vi "GeoData.vi"() -> ()   [LabVIEW 2017] (continued)
davenport\tNY\tDelaware County\tH1\n12468\t36025\tPrattsville\tNY\tDelaware County\tH1\n12760\t36025\tLong eddy\tNY\tDelaware County\tH1\n13820\t36025\tOneonta\tNY\tDelaware County\tH1\n13775\t36025\tFranklin\tNY\tDelaware County\tH1\n12430\t36025\tFleischmanns\tNY\tDelaware County\tH1\n12533\t36027\tHopewell junction\tNY\tDutchess County\tH1\n12545\t36027\tMillbrook\tNY\tDutchess County\tH1\n12583\t36027\tTivoli\tNY\tDutchess County\tH1\n12527\t36027\tGlenham\tNY\tDutchess County\tH1\n10512\t36027\tCarmel\tNY\tDutchess County\tH1\n12569\t36027\tPleasant valley\tNY\tDutchess County\tH1\n12601\t36027\tPoughkeepsie\tNY\tDutchess County\tH1\n12603\t36027\tPoughkeepsie\tNY\tDutchess County\tH1\n12511\t36027\tCastle point\tNY\tDutchess County\tH1\n12507\t36027\tBarrytown\tNY\tDutchess County\tH1\n12564\t36027\tPawling\tNY\tDutchess County\tH1\n12602\t36027\tPoughkeepsie\tNY\tDutchess County\tH1\n12531\t36027\tHolmes\tNY\tDutchess County\tH1\n12572\t36027\tRhinebeck\tNY\tDutchess County\tH1\n12538\t36027\tHyde park\tNY\tDutchess County\tH1\n12571\t36027\tRed hook\tNY\tDutchess County\tH1\n12594\t36027\tWingdale\tNY\tDutchess County\tH1\n12501\t36027\tAmenia\tNY\tDutchess County\tH1\n12570\t36027\tPoughquag\tNY\tDutchess County\tH1\n12581\t36027\tStanfordville\tNY\tDutchess County\tH1\n12582\t36027\tStormville\tNY\tDutchess County\tH1\n12590\t36027\tWappingers falls\tNY\tDutchess County\tH1\n12580\t36027\tStaatsburg\tNY\tDutchess County\tH1\n12546\t36027\tMillerton\tNY\tDutchess County\tH1\n12508\t36027\tBeacon\tNY\tDutchess County\tH1\n12540\t36027\tLagrangeville\tNY\tDutchess County\tH1\n12522\t36027\tDover plains\tNY\tDutchess County\tH1\n12504\t36027\tAnnandale on hudson\tNY\tDutchess County\tH1\n12537\t36027\tHughsonville\tNY\tDutchess County\tH1\n12574\t36027\tRhinecliff\tNY\tDutchess County\tH1\n12524\t36027\tFishkill\tNY\tDutchess County\tH1\n12585\t36027\tVerbank\tNY\tDutchess County\tH1\n12578\t36027\tSalt point\tNY\tDutchess County\tH1\n12567\t36027\tPine plains\tNY\tDutchess County\tH1\n12592\t36027\tWassaic\tNY\tDutchess County\tH1\n12514\t36027\tClinton corners\tNY\tDutchess County\tH1\n12506\t36027\tBangall\tNY\tDutchess County\tH1\n12512\t36027\tChelsea\tNY\tDutchess County\tH1\n12510\t36027\tBillings\tNY\tDutchess County\tH1\n12604\t36027\tPoughkeepsie\tNY\tDutchess County\tH1\n14052\t36029\tEast aurora\tNY\tErie County\tH1\n14036\t36029\tCorfu\tNY\tErie County\tH1\n14210\t36029\tBuffalo\tNY\tErie County\tH1\n14202\t36029\tBuffalo\tNY\tErie County\tH1\n14151\t36029\tTonawanda\tNY\tErie County\tH1\n14213\t36029\tBuffalo\tNY\tErie County\tH1\n14170\t36029\tWest falls\tNY\tErie County\tH1\n14219\t36029\tBuffalo\tNY\tErie County\tH1\n14223\t36029\tBuffalo\tNY\tErie County\tH1\n14085\t36029\tLake view\tNY\tErie County\tH1\n14080\t36029\tHolland\tNY\tErie County\tH1\n14134\t36029\tSardinia\tNY\tErie County\tH1\n14037\t36029\tCowlesville\tNY\tErie County\tH1\n14030\t36029\tChaffee\tNY\tErie County\tH1\n14241\t36029\tBuffalo\tNY\tErie County\tH1\n14059\t36029\tElma\tNY\tErie County\tH1\n14221\t36029\tBuffalo\tNY\tErie County\tH1\n14055\t36029\tEast concord\tNY\tErie County\tH1\n14272\t36029\tBuffalo\tNY\tErie County\tH1\n14140\t36029\tSpring brook\tNY\tErie County\tH1\n14075\t36029\tHamburg\tNY\tErie County\tH1\n14057\t36029\tEden\tNY\tErie County\tH1\n14208\t36029\tBuffalo\tNY\tErie County\tH1\n14214\t36029\tBuffalo\tNY\tErie County\tH1\n14206\t36029\tBuffalo\tNY\tErie County\tH1\n14139\t36029\tSouth wales\tNY\tErie County\tH1\n14209\t36029\tBuffalo\tNY\tErie County\tH1\n14225\t36029\tBuffalo\tNY\tErie County\tH1\n14025\t36029\tBoston\tNY\tErie County\tH1\n14260\t36029\tBuffalo\tNY\tErie County\tH1\n14263\t36029\tBuffalo\tNY\tErie County\tH1\n14027\t36029\tBrant\tNY\tErie County\tH1\n14110\t36029\tNorth boston\tNY\tErie County\tH1\n14032\t36029\tClarence center\tNY\tErie County\tH1\n14102\t36029\tMarilla\tNY\tErie County\tH1\n14091\t36029\tLawtons\tNY\tErie County\tH1\n14205\t36029\tBuffalo\tNY\tErie County\tH1\n14240\t36029\tBuffalo\tNY\tErie County\tH1\n14081\t36029\tIrving\tNY\tErie County\tH1\n14203\t36029\tBuffalo\tNY\tErie County\tH1\n14226\t36029\tBuffalo\tNY\tErie County\tH1\n14231\t36029\tBuffalo\tNY\tErie County\tH1\n14280\t36029\tBuffalo\tNY\tErie County\tH1\n14270\t36029\tBuffalo\tNY\tErie County\tH1\n14004\t36029\tAlden\tNY\tErie County\tH1\n14051\t36029\tEast amherst\tNY\tErie County\tH1\n14006\t36029\tAngola\tNY\tErie County\tH1\n14086\t36029\tLancaster\tNY\tErie County\tH1\n14127\t36029\tOrchard park\tNY\tErie County\tH1\n14150\t36029\tTonawanda\tNY\tErie County\tH1\n14211\t36029\tBuffalo\tNY\tErie County\tH1\n14227\t36029\tBuffalo\tNY\tErie County\tH1\n14228\t36029\tBuffalo\tNY\tErie County\tH1\n14070\t36029\tGowanda\tNY\tErie County\tH1\n14145\t36029\tStrykersville\tNY\tErie County\tH1\n14026\t36029\tBowmansville\tNY\tErie County\tH1\n14265\t36029\tBuffalo\tNY\tErie County\tH1\n14112\t36029\tNorth evans\tNY\tErie County\tH1\n14035\t36029\tCollins center\tNY\tErie County\tH1\n14233\t36029\tBuffalo\tNY\tErie County\tH1\n14043\t36029\tDepew\tNY\tErie County\tH1\n14212\t36029\tBuffalo\tNY\tErie County\tH1\n14169\t36029\tWales center\tNY\tErie County\tH1\n14269\t36029\tBuffalo\tNY\tErie County\tH1\n14072\t36029\tGrand island\tNY\tErie County\tH1\n14009\t36029\tArcade\tNY\tErie County\tH1\n14013\t36029\tBasom\tNY\tErie County\tH1\n14207\t36029\tBuffalo\tNY\tErie County\tH1\n14215\t36029\tBuffalo\tNY\tErie County\tH1\n14201\t36029\tBuffalo\tNY\tErie County\tH1\n14204\t36029\tBuffalo\tNY\tErie County\tH1\n14220\t36029\tBuffalo\tNY\tErie County\tH1\n14222\t36029\tBuffalo\tNY\tErie County\tH1\n14224\t36029\tBuffalo\tNY\tErie County\tH1\n14217\t36029\tBuffalo\tNY\tErie County\tH1\n14034\t36029\tCollins\tNY\tErie County\tH1\n14047\t36029\tDerby\tNY\tErie County\tH1\n14010\t36029\tAthol springs\tNY\tErie County\tH1\n14001\t36029\tAkron\tNY\tErie County\tH1\n14031\t36029\tClarence\tNY\tErie County\tH1\n14068\t36029\tGetzville\tNY\tErie County\tH1\n14111\t36029\tNorth collins\tNY\tErie County\tH1\n14216\t36029\tBuffalo\tNY\tErie County\tH1\n14141\t36029\tSpringville\tNY\tErie County\tH1\n14218\t36029\tBuffalo\tNY\tErie County\tH1\n14033\t36029\tColden\tNY\tErie County\tH1\n14069\t36029\tGlenwood\tNY\tErie County\tH1\n14061\t36029\tFarnham\tNY\tErie County\tH1\n14038\t36029\tCrittenden\tNY\tErie County\tH1\n14276\t36029\tBuffalo\tNY\tErie County\tH1\n14273\t36029\tBuffalo\tNY\tErie County\tH1\n12883\t36031\tTiconderoga\tNY\tEssex County\tH1\n12974\t36031\tPort henry\tNY\tEssex County\tH1\n12936\t36031\tEssex\tNY\tEssex County\tH1\n12996\t36031\tWillsboro\tNY\tEssex County\tH1\n12997\t36031\tWilmington\tNY\tEssex County\tH1\n12942\t36031\tKeene\tNY\tEssex County\tH1\n12998\t36031\tWitherbee\tNY\tEssex County\tH1\n12857\t36031\tOlmstedville\tNY\tEssex County\tH1\n12861\t36031\tPutnam station\tNY\tEssex County\tH1\n12956\t36031\tMineville\tNY\tEssex County\tH1\n12943\t36031\tKeene valley\tNY\tEssex County\tH1\n12983\t36031\tSaranac lake\tNY\tEssex County\tH1\n12993\t36031\tWestport\tNY\tEssex County\tH1\n12941\t36031\tJay\tNY\tEssex County\tH1\n12975\t36031\tPort kent\tNY\tEssex County\tH1\n12855\t36031\tNorth hudson\tNY\tEssex County\tH1\n12836\t36031\tHague\tNY\tEssex County\tH1\n12944\t36031\tKeeseville\tNY\tEssex County\tH1\n12987\t36031\tUpper jay\tNY\tEssex County\tH1\n12961\t36031\tMoriah center\tNY\tEssex County\tH1\n12870\t36031\tSchroon lake\tNY\tEssex County\tH1\n12972\t36031\tPeru\tNY\tEssex County\tH1\n12964\t36031\tNew russia\tNY\tEssex County\tH1\n12911\t36031\tKeeseville\tNY\tEssex County\tH1\n12879\t36031\tNewcomb\tNY\tEssex County\tH1\n12852\t36031\tNewcomb\tNY\tEssex County\tH1\n12946\t36031\tLake placid\tNY\tEssex County\tH1\n12853\t36031\tNorth creek\tNY\tEssex County\tH1\n12928\t36031\tCrown point\tNY\tEssex County\tH1\n12851\t36031\tMinerva\tNY\tEssex County\tH1\n12913\t36031\tBloomingdale\tNY\tEssex County\tH1\n12872\t36031\tSeverance\tNY\tEssex County\tH1\n12977\t36031\tRay brook\tNY\tEssex County\tH1\n12858\t36031\tParadox\tNY\tEssex County\tH1\n12950\t36031\tLewis\tNY\tEssex County\tH1\n12960\t36031\tMoriah\tNY\tEssex County\tH1\n12912\t36031\tAu sable forks\tNY\tEssex County\tH1\n12932\t36031\tElizabethtown\tNY\tEssex County\tH1\n12989\t36031\tVermontville\tNY\tEssex County\tH1\n12916\t36033\tBrushton\tNY\tFranklin County\tH1\n12981\t36033\tSaranac\tNY\tFranklin County\tH1\n12980\t36033\tSaint regis falls\tNY\tFranklin County\tH1\n12955\t36033\tLyon mountain\tNY\tFranklin County\tH1\n12976\t36033\tRainbow lake\tNY\tFranklin County\tH1\n12967\t36033\tNorth lawrence\tNY\tFranklin County\tH1\n12939\t36033\tGabriels\tNY\tFranklin County\tH1\n12926\t36033\tConstable\tNY\tFranklin County\tH1\n12937\t36033\tFort covington\tNY\tFranklin County\tH1\n12914\t36033\tBombay\tNY\tFranklin County\tH1\n12969\t36033\tOwls head\tNY\tFranklin County\tH1\n12953\t36033\tMalone\tNY\tFranklin County\tH1\n12983\t36033\tSaranac lake\tNY\tFranklin County\tH1\n13655\t36033\tHogansburg\tNY\tFranklin County\tH1\n12957\t36033\tMoira\tNY\tFranklin County\tH1\n12966\t36033\tNorth bangor\tNY\tFranklin County\tH1\n13683\t36033\tRooseveltown\tNY\tFranklin County\tH1\n12920\t36033\tChateaugay\tNY\tFranklin County\tH1\n12945\t36033\tLake clear\tNY\tFranklin County\tH1\n12970\t36033\tPaul smiths\tNY\tFranklin County\tH1\n12995\t36033\tWhippleville\tNY\tFranklin County\tH1\n12915\t36033\tBrainardsville\tNY\tFranklin County\tH1\n12930\t36033\tDickinson center\tNY\tFranklin County\tH1\n12913\t36033\tBloomingdale\tNY\tFranklin County\tH1\n12986\t36033\tTupper lake\tNY\tFranklin County\tH1\n12912\t36033\tAu sable forks\tNY\tFranklin County\tH1\n12917\t36033\tBurke\tNY\tFranklin County\tH1\n12989\t36033\tVermontville\tNY\tFranklin County\tH1\n12095\t36035\tJohnstown\tNY\tFulton County\tH1\n13329\t36035\tDolgeville\tNY\tFulton County\tH1\n12086\t36035\tHagaman\tNY\tFulton County\tH1\n12117\t36035\tMayfield\tNY\tFulton County\tH1\n12010\t36035\tAmsterdam\tNY\tFulton County\tH1\n12068\t36035\tFonda\tNY\tFulton County\tH1\n12032\t36035\tCaroga lake\tNY\tFulton County\tH1\n12025\t36035\tBroadalbin\tNY\tFulton County\tH1\n13452\t36035\tSaint johnsville\tNY\tFulton County\tH1\n13470\t36035\tStratford\tNY\tFulton County\tH1\n12070\t36035\tFort johnson\tNY\tFulton County\tH1\n13339\t36035\tFort plain\tNY\tFulton County\tH1\n12078\t36035\tGloversville\tNY\tFulton County\tH1\n12134\t36035\tNorthville\tNY\tFulton County\tH1\n13454\t36035\tSalisbury center\tNY\tFulton County\tH1\n14036\t36037\tCorfu\tNY\tGenesee County\tH1\n14525\t36037\tPavilion\tNY\tGenesee County\tH1\n14005\t36037\tAlexander\tNY\tGenesee County\tH1\n14428\t36037\tChurchville\tNY\tGenesee County\tH1\n14105\t36037\tMiddleport\tNY\tGenesee County\tH1\n14416\t36037\tBergen\tNY\tGenesee County\tH1\n14058\t36037\tElba\tNY\tGenesee County\tH1\n14422\t36037\tByron\tNY\tGenesee County\tH1\n14004\t36037\tAlden\tNY\tGenesee County\tH1\n14020\t36037\tBatavia\tNY\tGenesee County\tH1\n14591\t36037\tWyoming\tNY\tGenesee County\tH1\n14040\t36037\tDarien center\tNY\tGenesee County\tH1\n14557\t36037\tSouth byron\tNY\tGenesee County\tH1\n14103\t36037\tMedina\tNY\tGenesee County\tH1\n14054\t36037\tEast bethany\tNY\tGenesee County\tH1\n14056\t36037\tEast pembroke\tNY\tGenesee County\tH1\n14013\t36037\tBasom\tNY\tGenesee County\tH1\n14125\t36037\tOakfield\tNY\tGenesee County\tH1\n14143\t36037\tStafford\tNY\tGenesee County\tH1\n14482\t36037\tLe roy\tNY\tGenesee County\tH1\n14011\t36037\tAttica\tNY\tGenesee County\tH1\n14021\t36037\tBatavia\tNY\tGenesee County\tH1\n14001\t36037\tAkron\tNY\tGenesee County\tH1\n12413\t36039\tCairo\tNY\tGreene County\tH1\n12485\t36039\tTannersville\tNY\tGreene County\tH1\n12087\t36039\tHannacroix\tNY\tGreene County\tH1\n12450\t36039\tLanesville\tNY\tGreene County\tH1\n12454\t36039\tMaplecrest\tNY\tGreene County\tH1\n12051\t36039\tCoxsackie\tNY\tGreene County\tH1\n12407\t36039\tAshland\tNY\tGreene County\tH1\n12473\t36039\tRound top\tNY\tGreene County\tH1\n12469\t36039\tPreston hollow\tNY\tGreene County\tH1\n12192\t36039\tWest coxsackie\tNY\tGreene County\tH1\n12422\t36039\tDurham\tNY\tGreene County\tH1\n12460\t36039\tOak hill\tNY\tGreene County\tH1\n12015\t36039\tAthens\tNY\tGreene County\tH1\n12427\t36039\tElka park\tNY\tGreene County\tH1\n12176\t36039\tSurprise\tNY\tGreene County\tH1\n12444\t36039\tJewett\tNY\tGreene County\tH1\n12451\t36039\tLeeds\tNY\tGreene County\tH1\n12083\t36039\tGreenville\tNY\tGreene County\tH1\n12058\t36039\tEarlton\tNY\tGreene County\tH1\n12482\t36039\tSouth cairo\tNY\tGreene County\tH1\n12442\t36039\tHunter\tNY\tGreene County\tH1\n12124\t36039\tNew baltimore\tNY\tGreene County\tH1\n12414\t36039\tCatskill\tNY\tGreene County\tH1\n12480\t36039\tShandaken\tNY\tGreene County\tH1\n12042\t36039\tClimax\tNY\tGreene County\tH1\n12418\t36039\tCornwallville\tNY\tGreene County\tH1\n12436\t36039\tHaines falls\tNY\tGreene County\tH1\n12143\t36039\tRavena\tNY\tGreene County\tH1\n12120\t36039\tMedusa\tNY\tGreene County\tH1\n12431\t36039\tFreehold\tNY\tGreene County\tH1\n12492\t36039\tWest kill\tNY\tGreene County\tH1\n12463\t36039\tPalenville\tNY\tGreene County\tH1\n12468\t36039\tPrattsville\tNY\tGreene County\tH1\n12405\t36039\tAcra\tNY\tGreene County\tH1\n12439\t36039\tHensonville\tNY\tGreene County\tH1\n12423\t36039\tEast durham\tNY\tGreene County\tH1\n12430\t36039\tFleischmanns\tNY\tGreene County\tH1\n12470\t36039\tPurling\tNY\tGreene County\tH1\n12046\t36039\tCoeymans hollow\tNY\tGreene County\tH1\n12496\t36039\tWindham\tNY\tGreene County\tH1\n12424\t36039\tEast jewett\tNY\tGreene County\tH1\n12452\t36039\tLexington\tNY\tGreene County\tH1\n13353\t36041\tHoffmeister\tNY\tHamilton County\tH1\n13360\t36041\tInlet\tNY\tHamilton County\tH1\n12864\t36041\tSabael\tNY\tHamilton County\tH1\n12164\t36041\tSpeculator\tNY\tHamilton County\tH1\n12108\t36041\tLake pleasant\tNY\tHamilton County\tH1\n12190\t36041\tWells\tNY\tHamilton County\tH1\n12847\t36041\tLong lake\tNY\tHamilton County\tH1\n12032\t36041\tCaroga lake\tNY\tHamilton County\tH1\n12842\t36041\tIndian lake\tNY\tHamilton County\tH1\n12812\t36041\tBlue mountain lake\tNY\tHamilton County\tH1\n13331\t36041\tEagle bay\tNY\tHamilton County\tH1\n12139\t36041\tPiseco\tNY\tHamilton County\tH1\n12134\t36041\tNorthville\tNY\tHamilton County\tH1\n13436\t36041\tRaquette lake\tNY\tHamilton County\tH1\n13329\t36043\tDolgeville\tNY\tHerkimer County\tH1\n13406\t36043\tMiddleville\tNY\tHerkimer County\tH1\n13360\t36043\tInlet\tNY\tHerkimer County\tH1\n13338\t36043\tForestport\tNY\tHerkimer County\tH1\n13407\t36043\tMohawk\tNY\tHerkimer County\tH1\n13322\t36043\tClayville\tNY\tHerkimer County\tH1\n13420\t36043\tOld forge\tNY\tHerkimer County\tH1\n13413\t36043\tNew hartford\tNY\tHerkimer County\tH1\n13501\t36043\tUtica\tNY\tHerkimer County\tH1\n13361\t36043\tJordanville\tNY\tHerkimer County\tH1\n13340\t36043\tFrankfort\tNY\tHerkimer County\tH1\n13357\t36043\tIlion\tNY\tHerkimer County\tH1\n13456\t36043\tSauquoit\tNY\tHerkimer County\tH1\n13304\t36043\tBarneveld\tNY\tHerkimer County\tH1\n13367\t36043\tLowville\tNY\tHerkimer County\tH1\n13350\t36043\tHerkimer\tNY\tHerkimer County\tH1\n13324\t36043\tCold brook\tNY\tHerkimer County\tH1\n13438\t36043\tRemsen\tNY\tHerkimer County\tH1\n13491\t36043\tWest winfield\tNY\tHerkimer County\tH1\n13431\t36043\tPoland\tNY\tHerkimer County\tH1\n13439\t36043\tRichfield springs\tNY\tHerkimer County\tH1\n13470\t36043\tStratford\tNY\tHerkimer County\tH1\n13502\t36043\tUtica\tNY\tHerkimer County\tH1\n13416\t36043\tNewport\tNY\tHerkimer County\tH1\n13472\t36043\tThendara\tNY\tHerkimer County\tH1\n13339\t36043\tFort plain\tNY\tHerkimer County\tH1\n13365\t36043\tLittle falls\tNY\tHerkimer County\tH1\n13331\t36043\tEagle bay\tNY\tHerkimer County\tH1\n13454\t36043\tSalisbury center\tNY\tHerkimer County\tH1\n13475\t36043\tVan hornesville\tNY\tHerkimer County\tH1\n13145\t36045\tSandy creek\tNY\tJefferson County\tH1\n13601\t36045\tWatertown\tNY\tJefferson County\tH1\n13626\t36045\tCopenhagen\tNY\tJefferson County\tH1\n13619\t36045\tCarthage\tNY\tJefferson County\tH1\n13685\t36045\tSackets harbor\tNY\tJefferson County\tH1\n13636\t36045\tEllisburg\tNY\tJefferson County\tH1\n13671\t36045\tAntwerp\tNY\tJefferson County\tH1\n13693\t36045\tThree mile bay\tNY\tJefferson County\tH1\n13682\t36045\tRodman\tNY\tJefferson County\tH1\n13673\t36045\tPhiladelphia\tNY\tJefferson County\tH1\n13691\t36045\tTheresa\tNY\tJefferson County\tH1\n13606\t36045\tAdams center\tNY\tJefferson County\tH1\n13607\t36045\tAlexandria bay\tNY\tJefferson County\tH1\n13631\t36045\tDenmark\tNY\tJefferson County\tH1\n13622\t36045\tChaumont\tNY\tJefferson County\tH1\n13692\t36045\tThousand island park\tNY\tJefferson County\tH1\n13624\t36045\tClayton\tNY\tJefferson County\tH1\n13616\t36045\tCalcium\tNY\tJefferson County\tH1\n13675\t36045\tPlessis\tNY\tJefferson County\tH1\n13661\t36045\tMannsville\tNY\tJefferson County\tH1\n13602\t36045\tFort drum\tNY\tJefferson County\tH1\n13651\t36045\tHenderson harbor\tNY\tJefferson County\tH1\n13632\t36045\tDepauville\tNY\tJefferson County\tH1\n13615\t36045\tBrownville\tNY\tJefferson County\tH1\n13611\t36045\tBelleville\tNY\tJefferson County\tH1\n13641\t36045\tFishers landing\tNY\tJefferson County\tH1\n13608\t36045\tAntwerp\tNY\tJefferson County\tH1\n13618\t36045\tCape vincent\tNY\tJefferson County\tH1\n13656\t36045\tLa fargeville\tNY\tJefferson County\tH1\n13659\t36045\tLorraine\tNY\tJefferson County\tH1\n13646\t36045\tHammond\tNY\tJefferson County\tH1\n13638\t36045\tFelts mills\tNY\tJefferson County\tH1\n13665\t36045\tNatural bridge\tNY\tJefferson County\tH1\n13634\t36045\tDexter\tNY\tJefferson County\tH1\n13605\t36045\tAdams\tNY\tJefferson County\tH1\n13637\t36045\tEvans mills\tNY\tJefferson County\tH1\n13612\t36045\tBlack river\tNY\tJefferson County\tH1\n13640\t36045\tWellesley island\tNY\tJefferson County\tH1\n13603\t36045\tWatertown\tNY\tJefferson County\tH1\n13642\t36045\tGouverneur\tNY\tJefferson County\tH1\n13650\t36045\tHenderson\tNY\tJefferson County\tH1\n13679\t36045\tRedwood\tNY\tJefferson County\tH1\n13083\t36045\tLacona\tNY\tJefferson County\tH1\n13628\t36045\tDeferiet\tNY\tJefferson County\tH1\n13643\t36045\tGreat bend\tNY\tJefferson County\tH1\n13674\t36045\tPierrepont manor\tNY\tJefferson County\tH1\n11202\t36047\tBrooklyn\tNY\tKings County\tH6\n11204\t36047\tBrooklyn\tNY\tKings County\tH6\n11203\t36047\tBrooklyn\tNY\tKings County\tH6\n11210\t36047\tBrooklyn\tNY\tKings County\tH6\n11213\t36047\tBrooklyn\tNY\tKings County\tH6\n11216\t36047\tBrooklyn\tNY\tKings County\tH6\n11229\t36047\tBrooklyn\tNY\tKings County\tH6\n11225\t36047\tBrooklyn\tNY\tKings County\tH6\n11238\t36047\tBrooklyn\tNY\tKings County\tH6\n11239\t36047\tBrooklyn\tNY\tKings County\tH6\n11211\t36047\tBrooklyn\tNY\tKings County\tH6\n11223\t36047\tBrooklyn\tNY\tKings County\tH6\n11228\t36047\tBrooklyn\tNY\tKings County\tH6\n11417\t36047\tOzone park\tNY\tKings County\tH6\n11242\t36047\tBrooklyn\tNY\tKings County\tH6\n11205\t36047\tBrooklyn\tNY\tKings County\tH6\n11208\t36047\tBrooklyn\tNY\tKings County\tH6\n11212\t36047\tBrooklyn\tNY\tKings County\tH6\n11233\t36047\tBrooklyn\tNY\tKings County\tH6\n11245\t36047\tBrooklyn\tNY\tKings County\tH6\n11206\t36047\tBrooklyn\tNY\tKings County\tH6\n11235\t36047\tBrooklyn\tNY\tKings County\tH6\n11414\t36047\tHoward beach\tNY\tKings County\tH6\n11251\t36047\tBrooklyn\tNY\tKings County\tH6\n11220\t36047\tBrooklyn\tNY\tKings County\tH6\n11247\t36047\tBrooklyn\tNY\tKings County\tH6\n11219\t36047\tBrooklyn\tNY\tKings County\tH6\n11232\t36047\tBrooklyn\tNY\tKings County\tH6\n11236\t36047\tBrooklyn\tNY\tKings County\tH6\n11209\t36047\tBrooklyn\tNY\tKings County\tH6\n11215\t36047\tBrooklyn\tNY\tKings County\tH6\n11214\t36047\tBrooklyn\tNY\tKings County\tH6\n11221\t36047\tBrooklyn\tNY\tKings County\tH6\n11230\t36047\tBrooklyn\tNY\tKings County\tH6\n11234\t36047\tBrooklyn\tNY\tKings County\tH6\n11249\t36047\tBrooklyn\tNY\tKings County\tH6\n11421\t36047\tWoodhaven\tNY\tKings County\tH6\n11243\t36047\tBrooklyn\tNY\tKings County\tH6\n11252\t36047\tBrooklyn\tNY\tKings County\tH6\n11201\t36047\tBrooklyn\tNY\tKings County\tH6\n11207\t36047\tBrooklyn\tNY\tKings County\tH6\n11218\t36047\tBrooklyn\tNY\tKings County\tH6\n11217\t36047\tBrooklyn\tNY\tKings County\tH6\n11224\t36047\tBrooklyn\tNY\tKings County\tH6\n11222\t36047\tBrooklyn\tNY\tKings County\tH6\n11226\t36047\tBrooklyn\tNY\tKings County\tH6\n11231\t36047\tBrooklyn\tNY\tKings County\tH6\n11237\t36047\tBrooklyn\tNY\tKings County\tH6\n11256\t36047\tBrooklyn\tNY\tKings County\tH6\n11416\t36047\tOzone park\tNY\tKings County\tH6\n11241\t36047\tBrooklyn\tNY\tKings County\tH6\n13473\t36049\tTurin\tNY\tLewis County\tH1\n13601\t36049\tWatertown\tNY\tLewis County\tH1\n13626\t36049\tCopenhagen\tNY\tLewis County\tH1\n13619\t36049\tCarthage\tNY\tLewis County\tH1\n13620\t36049\tCastorland\tNY\tLewis County\tH1\n13682\t36049\tRodman\tNY\tLewis County\tH1\n13312\t36049\tBrantingham\tNY\tLewis County\tH1\n13343\t36049\tGlenfield\tNY\tLewis County\tH1\n13368\t36049\tLyons falls\tNY\tLewis County\tH1\n13345\t36049\tGreig\tNY\tLewis County\tH1\n13493\t36049\tWilliamstown\tNY\tLewis County\tH1\n13367\t36049\tLowville\tNY\tLewis County\tH1\n13327\t36049\tCroghan\tNY\tLewis County\tH1\n13433\t36049\tPort leyden\tNY\tLewis County\tH1\n13437\t36049\tRedfield\tNY\tLewis County\tH1\n13648\t36049\tHarrisville\tNY\tLewis County\tH1\n13305\t36049\tBeaver falls\tNY\tLewis County\tH1\n13471\t36049\tTaberg\tNY\tLewis County\tH1\n13665\t36049\tNatural bridge\tNY\tLewis County\tH1\n13309\t36049\tBoonville\tNY\tLewis County\tH1\n13316\t36049\tCamden\tNY\tLewis County\tH1\n13404\t36049\tMartinsburg\tNY\tLewis County\tH1\n13489\t36049\tWest leyden\tNY\tLewis County\tH1\n13325\t36049\tConstableville\tNY\tLewis County\tH1\n14525\t36051\tPavilion\tNY\tLivingston County\tH1\n14592\t36051\tYork\tNY\tLivingston County\tH1\n14558\t36051\tSouth lima\tNY\tLivingston County\tH1\n14454\t36051\tGeneseo\tNY\tLivingston County\tH1\n14512\t36051\tNaples\tNY\tLivingston County\tH1\n14822\t36051\tCanaseraga\tNY\tLivingston County\tH1\n14836\t36051\tDalton\tNY\tLivingston County\tH1\n14486\t36051\tLinwood\tNY\tLivingston County\tH1\n14472\t36051\tHoneoye falls\tNY\tLivingston County\tH1\n14884\t36051\tSwain\tNY\tLivingston County\tH1\n14488\t36051\tLivonia center\tNY\tLivingston County\tH1\n14480\t36051\tLakeville\tNY\tLivingston County\tH1\n14560\t36051\tSpringwater\tNY\tLivingston County\tH1\n14510\t36051\tMount morris\tNY\tLivingston County\tH1\n14545\t36051\tScottsburg\tNY\tLivingston County\tH1\n14437\t36051\tDansville\tNY\tLivingston County\tH1\n14517\t36051\tNunda\tNY\tLivingston County\tH1\n14533\t36051\tPiffard\tNY\tLivingston County\tH1\n14556\t36051\tSonyea\tNY\tLivingston County\tH1\n14539\t36051\tRetsof\tNY\tLivingston County\tH1\n14435\t36051\tConesus\tNY\tLivingston County\tH1\n14485\t36051\tLima\tNY\tLivingston County\tH1\n14487\t36051\tLivonia\tNY\tLivingston County\tH1\n14466\t36051\tHemlock\tNY\tLivingston County\tH1\n14481\t36051\tLeicester\tNY\tLivingston County\tH1\n14846\t36051\tHunt\tNY\tLivingston County\tH1\n14482\t36051\tLe roy\tNY\tLivingston County\tH1\n14471\t36051\tHoneoye\tNY\tLivingston County\tH1\n14572\t36051\tWayland\tNY\tLivingston County\tH1\n14546\t36051\tScottsville\tNY\tLivingston County\tH1\n14414\t36051\tAvon\tNY\tLivingston County\tH1\n14530\t36051\tPerry\tNY\tLivingston County\tH1\n14462\t36051\tGroveland\tNY\tLivingston County\tH1\n14423\t36051\tCaledonia\tNY\tLivingston County\tH1\n13035\t36053\tCazenovia\tNY\tMadison County\tH1\n13408\t36053\tMorrisville\tNY\tMadison County\tH1\n13163\t36053\tWampsville\tNY\tMadison County\tH1\n13355\t36053\tHubbardsville\tNY\tMadison County\tH1\n13032\t36053\tCanastota\tNY\tMadison County\tH1\n13460\t36053\tSherburne\tNY\tMadison County\tH1\n13030\t36053\tBridgeport\tNY\tMadison County\tH1\n13418\t36053\tNorth brookfield\tNY\tMadison County\tH1\n13364\t36053\tLeonardsville\tNY\tMadison County\tH1\n13122\t36053\tNew woodstock\tNY\tMadison County\tH1\n13491\t36053\tWest winfield\tNY\tMadison County\tH1\n13485\t36053\tWest edmeston\tNY\tMadison County\tH1\n13484\t36053\tWest eaton\tNY\tMadison County\tH1\n13037\t36053\tChittenango\tNY\tMadison County\tH1\n13104\t36053\tManlius\tNY\tMadison County\tH1\n13052\t36053\tDe ruyter\tNY\tMadison County\tH1\n13072\t36053\tGeorgetown\tNY\tMadison County\tH1\n13061\t36053\tErieville\tNY\tMadison County\tH1\n13409\t36053\tMunnsville\tNY\tMadison County\tH1\n13332\t36053\tEarlville\tNY\tMadison County\tH1\n13334\t36053\tEaton\tNY\tMadison County\tH1\n13464\t36053\tSmyrna\tNY\tMadison County\tH1\n13134\t36053\tPeterboro\tNY\tMadison County\tH1\n13402\t36053\tMadison\tNY\tMadison County\tH1\n13480\t36053\tWaterville\tNY\tMadison County\tH1\n13310\t36053\tBouckville\tNY\tMadison County\tH1\n13425\t36053\tOriskany falls\tNY\tMadison County\tH1\n13043\t36053\tClockville\tNY\tMadison County\tH1\n13082\t36053\tKirkville\tNY\tMadison County\tH1\n13346\t36053\tHamilton\tNY\tMadison County\tH1\n13421\t36053\tOneida\tNY\tMadison County\tH1\n13314\t36053\tBrookfield\tNY\tMadison County\tH1\n14464\t36055\tHamlin\tNY\tMonroe County\tH1\n14476\t36055\tKendall\tNY\tMonroe County\tH1\n14580\t36055\tWebster\tNY\tMonroe County\tH1\n14604\t36055\tRochester\tNY\tMonroe County\tH1\n14692\t36055\tRochester\tNY\tMonroe County\tH1\n14651\t36055\tRochester\tNY\tMonroe County\tH1\n14646\t36055\tRochester\tNY\tMonroe County\tH1\n14502\t36055\tMacedon\tNY\tMonroe County\tH1\n14603\t36055\tRochester\tNY\tMonroe County\tH1\n14609\t36055\tRochester\tNY\tMonroe County\tH1\n14610\t36055\tRochester\tNY\tMonroe County\tH1\n14608\t36055\tRochester\tNY\tMonroe County\tH1\n14621\t36055\tRochester\tNY\tMonroe County\tH1\n14428\t36055\tChurchville\tNY\tMonroe County\tH1\n14514\t36055\tNorth chili\tNY\tMonroe County\tH1\n14508\t36055\tMorton\tNY\tMonroe County\tH1\n14515\t36055\tNorth greece\tNY\tMonroe County\tH1\n14410\t36055\tAdams basin\tNY\tMonroe County\tH1\n14420\t36055\tBrockport\tNY\tMonroe County\tH1\n14416\t36055\tBergen\tNY\tMonroe County\tH1\n14534\t36055\tPittsford\tNY\tMonroe County\tH1\n14519\t36055\tOntario\tNY\tMonroe County\tH1\n14526\t36055\tPenfield\tNY\tMonroe County\tH1\n14472\t36055\tHoneoye falls\tNY\tMonroe County\tH1\n14626\t36055\tRochester\tNY\tMonroe County\tH1\n14430\t36055\tClarkson\tNY\tMonroe County\tH1\n14649\t36055\tRochester\tNY\tMonroe County\tH1\n14643\t36055\tRochester\tNY\tMonroe County\tH1\n14639\t36055\tRochester\tNY\tMonroe County\tH1\n14450\t36055\tFairport\tNY\tMonroe County\tH1\n14606\t36055\tRochester\tNY\tMonroe County\tH1\n14607\t36055\tRochester\tNY\tMonroe County\tH1\n14614\t36055\tRochester\tNY\tMonroe County\tH1\n14619\t36055\tRochester\tNY\tMonroe County\tH1\n14613\t36055\tRochester\tNY\tMonroe County\tH1\n14602\t36055\tRochester\tNY\tMonroe County\tH1\n14647\t36055\tRochester\tNY\tMonroe County\tH1\n14468\t36055\tHilton\tNY\tMonroe County\tH1\n14611\t36055\tRochester\tNY\tMonroe County\tH1\n14623\t36055\tRochester\tNY\tMonroe County\tH1\n14624\t36055\tRochester\tNY\tMonroe County\tH1\n14625\t36055\tRochester\tNY\tMonroe County\tH1\n14622\t36055\tRochester\tNY\tMonroe County\tH1\n14638\t36055\tRochester\tNY\tMonroe County\tH1\n14467\t36055\tHenrietta\tNY\tMonroe County\tH1\n14564\t36055\tVictor\tNY\tMonroe County\tH1\n14605\t36055\tRochester\tNY\tMonroe County\tH1\n14559\t36055\tSpencerport\tNY\tMonroe County\tH1\n14586\t36055\tWest henrietta\tNY\tMonroe County\tH1\n14612\t36055\tRochester\tNY\tMonroe County\tH1\n14615\t36055\tRochester\tNY\tMonroe County\tH1\n14618\t36055\tRochester\tNY\tMonroe County\tH1\n14620\t36055\tRochester\tNY\tMonroe County\tH1\n14511\t36055\tMumford\tNY\tMonroe County\tH1\n14642\t36055\tRochester\tNY\tMonroe County\tH1\n14650\t36055\tRochester\tNY\tMonroe County\tH1\n14627\t36055\tRochester\tNY\tMonroe County\tH1\n14482\t36055\tLe roy\tNY\tMonroe County\tH1\n14506\t36055\tMendon\tNY\tMonroe County\tH1\n14470\t36055\tHolley\tNY\tMonroe County\tH1\n14616\t36055\tRochester\tNY\tMonroe County\tH1\n14617\t36055\tRochester\tNY\tMonroe County\tH1\n14546\t36055\tScottsville\tNY\tMonroe County\tH1\n14652\t36055\tRochester\tNY\tMonroe County\tH1\n14414\t36055\tAvon\tNY\tMonroe County\tH1\n14445\t36055\tEast rochester\tNY\tMonroe County\tH1\n14543\t36055\tRush\tNY\tMonroe County\tH1\n14423\t36055\tCaledonia\tNY\tMonroe County\tH1\n14653\t36055\tRochester\tNY\tMonroe County\tH1\n12095\t36057\tJohnstown\tNY\tMontgomery County\tH1\n12086\t36057\tHagaman\tNY\tMontgomery County\tH1\n12137\t36057\tPattersonville\tNY\tMontgomery County\tH1\n13320\t36057\tCherry valley\tNY\tMontgomery County\tH1\n12010\t36057\tAmsterdam\tNY\tMontgomery County\tH1\n12053\t36057\tDelanson\tNY\tMontgomery County\tH1\n13459\t36057\tSharon springs\tNY\tMontgomery County\tH1\n12160\t36057\tSloansville\tNY\tMontgomery County\tH1\n12177\t36057\tTribes hill\tNY\tMontgomery County\tH1\n12072\t36057\tFultonville\tNY\tMontgomery County\tH1\n12068\t36057\tFonda\tNY\tMontgomery County\tH1\n12066\t36057\tEsperance\tNY\tMontgomery County\tH1\n12166\t36057\tSprakers\tNY\tMontgomery County\tH1\n13317\t36057\tCanajoharie\tNY\tMontgomery County\tH1\n13410\t36057\tNelliston\tNY\tMontgomery County\tH1\n13428\t36057\tPalatine bridge\tNY\tMontgomery County\tH1\n13452\t36057\tSaint johnsville\tNY\tMontgomery County\tH1\n12070\t36057\tFort johnson\tNY\tMontgomery County\tH1\n13339\t36057\tFort plain\tNY\tMontgomery County\tH1\n12069\t36057\tFort hunter\tNY\tMontgomery County\tH1\n11001\t36059\tFloral park\tNY\tNassau County\tH1\n11520\t36059\tFreeport\tNY\tNassau County\tH1\n11550\t36059\tHempstead\tNY\tNassau County\tH1\n11553\t36059\tUniondale\tNY\tNassau County\tH1\n11565\t36059\tMalverne\tNY\tNassau County\tH1\n11545\t36059\tGlen head\tNY\tNassau County\tH1\n11581\t36059\tValley stream\tNY\tNassau County\tH1\n11732\t36059\tEast norwich\tNY\tNassau County\tH1\n11771\t36059\tOyster bay\tNY\tNassau County\tH1\n11783\t36059\tSeaford\tNY\tNassau County\tH1\n11791\t36059\tSyosset\tNY\tNassau County\tH1\n11531\t36059\tGarden city\tNY\tNassau County\tH1\n11020\t36059\tGreat neck\tNY\tNassau County\tH1\n11050\t36059\tPort washington\tNY\tNassau County\tH1\n11501\t36059\tMineola\tNY\tNassau County\tH1\n11566\t36059\tMerrick\tNY\tNassau County\tH1\n11552\t36059\tWest hempstead\tNY\tNassau County\tH1\n11598\t36059\tWoodmere\tNY\tNassau County\tH1\n11575\t36059\tRoosevelt\tNY\tNassau County\tH1\n11735\t36059\tFarmingdale\tNY\tNassau County\tH1\n11801\t36059\tHicksville\tNY\tNassau County\tH1\n11803\t36059\tPlainview\tNY\tNassau County\tH1\n11509\t36059\tAtlantic beach\tNY\tNassau County\tH1\n11002\t36059\tFloral park\tNY\tNassau County\tH1\n11802\t36059\tHicksville\tNY\tNassau County\tH1\n11547\t36059\tGlenwood landing\tNY\tNassau County\tH1\n11753\t36059\tJericho\tNY\tNassau County\tH1\n11758\t36059\tMassapequa\tNY\tNassau County\tH1\n11568\t36059\tOld westbury\tNY\tNassau County\tH1\n11815\t36059\tHicksville\tNY\tNassau County\tH1\n11551\t36059\tHempstead\tNY\tNassau County\tH1\n11558\t36059\tIsland park\tNY\tNassau County\tH1\n11549\t36059\tHempstead\tNY\tNassau County\tH1\n11580\t36059\tValley stream\tNY\tNassau County\tH1\n11570\t36059\tRockville centre\tNY\tNassau County\tH1\n11579\t36059\tSea cliff\tNY\tNassau County\tH1\n11710\t36059\tBellmore\tNY\tNassau County\tH1\n11709\t36059\tBayville\tNY\tNassau County\tH1\n11793\t36059\tWantagh\tNY\tNassau County\tH1\n11096\t36059\tInwood\tNY\tNassau County\tH1\n11582\t36059\tValley stream\tNY\tNassau County\tH1\n11765\t36059\tMill neck\tNY\tNassau County\tH1\n11024\t36059\tGreat neck\tNY\tNassau County\tH1\n11530\t36059\tGarden city\tNY\tNassau County\tH1\n11559\t36059\tLawrence\tNY\tNassau County\tH1\n11548\t36059\tGreenvale\tNY\tNassau County\tH1\n11701\t36059\tAmityville\tNY\tNassau County\tH1\n11571\t36059\tRockville centre\tNY\tNassau County\tH1\n11762\t36059\tMassapequa park\tNY\tNassau County\tH1\n11023\t36059\tGreat neck\tNY\tNassau County\tH1\n11003\t36059\tElmont\tNY\tNassau County\tH1\n11010\t36059\tFranklin square\tNY\tNassau County\tH1\n11561\t36059\tLong beach\tNY\tNassau County\tH1\n11557\t36059\tHewlett\tNY\tNassau County\tH1\n11572\t36059\tOceanside\tNY\tNassau County\tH1\n11576\t36059\tRoslyn\tNY\tNassau County\tH1\n11756\t36059\tLevittown\tNY\tNassau County\tH1\n11804\t36059\tOld bethpage\tNY\tNassau County\tH1\n11005\t36059\tFloral park\tNY\tNassau County\tH1\n11022\t36059\tGreat neck\tNY\tNassau County\tH1\n11724\t36059\tCold spring harbor\tNY\tNassau County\tH1\n11556\t36059\tUniondale\tNY\tNassau County\tH1\n11599\t36059\tGarden city\tNY\tNassau County\tH1\n11040\t36059\tNew hyde park\tNY\tNassau County\tH1\n11021\t36059\tGreat neck\tNY\tNassau County\tH1\n11030\t36059\tManhasset\tNY\tNassau County\tH1\n11518\t36059\tEast rockaway\tNY\tNassau County\tH1\n11507\t36059\tAlbertson\tNY\tNassau County\tH1\n11590\t36059\tWestbury\tNY\tNassau County\tH1\n11714\t36059\tBethpage\tNY\tNassau County\tH1\n11797\t36059\tWoodbury\tNY\tNassau County\tH1\n11042\t36059\tNew hyde park\tNY\tNassau County\tH1\n11514\t36059\tCarle place\tNY\tNassau County\tH1\n11542\t36059\tGlen cove\tNY\tNassau County\tH1\n11510\t36059\tBaldwin\tNY\tNassau County\tH1\n11516\t36059\tCedarhurst\tNY\tNassau County\tH1\n11554\t36059\tEast meadow\tNY\tNassau County\tH1\n11563\t36059\tLynbrook\tNY\tNassau County\tH1\n11560\t36059\tLocust valley\tNY\tNassau County\tH1\n11577\t36059\tRoslyn heights\tNY\tNassau County\tH1\n11596\t36059\tWilliston park\tNY\tNassau County\tH1\n11569\t36059\tPoint lookout\tNY\tNassau County\tH1\n11773\t36059\tMelville\tNY\tNassau County\tH1\n10025\t36061\tNew york\tNY\tNew York County\tH6\n10075\t36061\tNew york\tNY\tNew York County\tH6\n10036\t36061\tNew york\tNY\tNew York County\tH6\n10282\t36061\tNew york\tNY\tNew York County\tH6\n10271\t36061\tNew york\tNY\tNew York County\tH6\n10155\t36061\tNew york\tNY\tNew York County\tH6\n10279\t36061\tNew york\tNY\tNew York County\tH6\n10174\t36061\tNew york\tNY\tNew York County\tH6\n10112\t36061\tNew york\tNY\tNew York County\tH6\n10178\t36061\tNew york\tNY\tNew York County\tH6\n10179\t36061\tNew york\tNY\tNew York County\tH6\n10080\t36061\tNew york\tNY\tNew York County\tH6\n10014\t36061\tNew york\tNY\tNew York County\tH6\n10024\t36061\tNew york\tNY\tNew York County\tH6\n10027\t36061\tNew york\tNY\tNew York County\tH6\n10030\t36061\tNew york\tNY\tNew York County\tH6\n10032\t36061\tNew york\tNY\tNew York County\tH6\n10165\t36061\tNew york\tNY\tNew York County\tH6\n10123\t36061\tNew york\tNY\tNew York County\tH6\n10122\t36061\tNew york\tNY\tNew York County\tH6\n10158\t36061\tNew york\tNY\tNew York County\tH6\n10133\t36061\tNew york\tNY\tNew York County\tH6\n10277\t36061\tNew york\tNY\tNew York County\tH6\n10203\t36061\tNew york\tNY\tNew York County\tH6\n10005\t36061\tNew york\tNY\tNew York County\tH6\n10009\t36061\tNew york\tNY\tNew York County\tH6\n10029\t36061\tNew york\tNY\tNew York County\tH6\n10034\t36061\tNew york\tNY\tNew York County\tH6\n10065\t36061\tNew york\tNY\tNew York County\tH6\n10044\t36061\tNew york\tNY\tNew York County\tH6\n10176\t36061\tNew york\tNY\tNew York County\tH6\n10169\t36061\tNew york\tNY\tNew York County\tH6\n10104\t36061\tNew york\tNY\tNew York County\tH6\n10115\t36061\tNew york\tNY\tNew York County\tH6\n10151\t36061\tNew york\tNY\tNew York County\tH6\n10274\t36061\tNew york\tNY\tNew York County\tH6\n10171\t36061\tNew york\tNY\tNew York County\tH6\n10045\t36061\tNew york\tNY\tNew York County\tH6\n10125\t36061\tNew york\tNY\tNew York County\tH6\n10211\t36061\tNew york\tNY\tNew York County\tH6\n10081\t36061\tNew york\tNY\tNew York County\tH6\n10130\t36061\tNew york\tNY\tNew York County\tH6\n10004\t36061\tNew york\tNY\tNew York County\tH6\n10003\t36061\tNew york\tNY\tNew York County\tH6\n10007\t36061\tNew york\tNY\tNew York County\tH6\n10022\t36061\tNew york\tNY\tNew York County\tH6\n10026\t36061\tNew york\tNY\tNew York County\tH6\n10033\t36061\tNew york\tNY\tNew York County\tH6\n10175\t36061\tNew york\tNY\tNew York County\tH6\n10163\t36061\tNew york\tNY\tNew York County\tH6\n10156\t36061\tNew york\tNY\tNew York County\tH6\n10463\t36061\tBronx\tNY\tNew York County\tH6\n10008\t36061\tNew york\tNY\tNew York County\tH6\n10111\t36061\tNew york\tNY\tNew York County\tH6\n10108\t36061\tNew york\tNY\tNew York County\tH6\n10138\t36061\tNew york\tNY\tNew York County\tH6\n10002\t36061\tNew york\tNY\tNew York County\tH6\n10020\t36061\tNew york\tNY\tNew York County\tH6\n10028\t36061\tNew york\tNY\tNew York County\tH6\n10069\t36061\tNew york\tNY\tNew York County\tH6\n10119\t36061\tNew york\tNY\tNew York County\tH6\n10038\t36061\tNew york\tNY\tNew York County\tH6\n10129\t36061\tNew york\tNY\tNew York County\tH6\n10110\t36061\tNew york\tNY\tNew York County\tH6\n10101\t36061\tNew york\tNY\tNew York County\tH6\n10281\t36061\tNew york\tNY\tNew York County\tH6\n10199\t36061\tNew york\tNY\tNew York County\tH6\n10103\t36061\tNew york\tNY\tNew York County\tH6\n10173\t36061\tNew york\tNY\tNew York County\tH6\n10055\t36061\tNew york\tNY\tNew York County\tH6\n10117\t36061\tNew york\tNY\tNew York County\tH6\n10160\t36061\tNew york\tNY\tNew York County\tH6\n10275\t36061\tNew york\tNY\tNew York County\tH6\n10131\t36061\tNew york\tNY\tNew York County\tH6\n10006\t36061\tNew york\tNY\tNew York County\tH6\n10012\t36061\tNew york\tNY\tNew York County\tH6\n10040\t36061\tNew york\tNY\tNew York County\tH6\n10039\t36061\tNew york\tNY\tNew York County\tH6\n10185\t36061\tNew york\tNY\tNew York County\tH6\n10258\t36061\tNew york\tNY\tNew York County\tH6\n10170\t36061\tNew york\tNY\tNew York County\tH6\n10107\t36061\tNew york\tNY\tNew York County\tH6\n10153\t36061\tNew york\tNY\tNew York County\tH6\n10268\t36061\tNew york\tNY\tNew York County\tH6\n10159\t36061\tNew york\tNY\tNew York County\tH6\n10167\t36061\tNew york\tNY\tNew York County\tH6\n10126\t36061\tNew york\tNY\tNew York County\tH6\n10043\t36061\tNew york\tNY\tNew York County\tH6\n10010\t36061\tNew york\tNY\tNew York County\tH6\n10013\t36061\tNew york\tNY\tNew York County\tH6\n10016\t36061\tNew york\tNY\tNew York County\tH6\n10035\t36061\tNew york\tNY\tNew York County\tH6\n10037\t36061\tNew york\tNY\tNew York County\tH6\n10166\t36061\tNew york\tNY\tNew York County\tH6\n10278\t36061\tNew york\tNY\tNew York County\tH6\n10105\t36061\tNew york\tNY\tNew York County\tH6\n10041\t36061\tNew york\tNY\tNew York County\tH6\n10272\t36061\tNew york\tNY\tNew York County\tH6\n10154\t36061\tNew york\tNY\tNew York County\tH6\n10120\t36061\tNew york\tNY\tNew York County\tH6\n10150\t36061\tNew york\tNY\tNew York County\tH6\n10164\t36061\tNew york\tNY\tNew York County\tH6\n10285\t36061\tNew york\tNY\tNew York County\tH6\n10212\t36061\tNew york\tNY\tNew York County\tH6\n10001\t36061\tNew york\tNY\tNew York County\tH6\n10011\t36061\tNew york\tNY\tNew York County\tH6\n10017\t36061\tNew york\tNY\tNew York County\tH6\n10021\t36061\tNew york\tNY\tNew York County\tH6\n10019\t36061\tNew york\tNY\tNew York County\tH6\n10018\t36061\tNew york\tNY\tNew York County\tH6\n10023\t36061\tNew york\tNY\tNew York County\tH6\n10031\t36061\tNew york\tNY\tNew York County\tH6\n10118\t36061\tNew york\tNY\tNew York County\tH6\n10128\t36061\tNew york\tNY\tNew York County\tH6\n10280\t36061\tNew york\tNY\tNew York County\tH6\n10113\t36061\tNew york\tNY\tNew York County\tH6\n10116\t36061\tNew york\tNY\tNew York County\tH6\n10168\t36061\tNew york\tNY\tNew York County\tH6\n10121\t36061\tNew york\tNY\tNew York County\tH6\n10152\t36061\tNew york\tNY\tNew York County\tH6\n10276\t36061\tNew york\tNY\tNew York County\tH6\n10162\t36061\tNew york\tNY\tNew York County\tH6\n10177\t36061\tNew york\tNY\tNew York County\tH6\n10172\t36061\tNew york\tNY\tNew York County\tH6\n10124\t36061\tNew york\tNY\tNew York County\tH6\n10106\t36061\tNew york\tNY\tNew York County\tH6\n10213\t36061\tNew york\tNY\tNew York County\tH6\n10269\t36061\tNew york\tNY\tNew York County\tH6\n10157\t36061\tNew york\tNY\tNew York County\tH6\n14109\t36063\tNiagara university\tNY\tNiagara County\tH1\n14126\t36063\tOlcott\tNY\tNiagara County\tH1\n14094\t36063\tLockport\tNY\tNiagara County\tH1\n14105\t36063\tMiddleport\tNY\tNiagara County\tH1\n14172\t36063\tWilson\tNY\t
